vi "GenerateDGMLOwnerlessFilesFolderString.vi"(8 "Links in":T1, 9 "Nodes in":T1, 10 "ILabVIEWItem in":refnum<class "ILabVIEWItem.lvclass">, 11 "CGrapherDGML in":refnum<class "CGrapherDGML.lvclass">) -> (0 "Links":T1, 1 "Nodes":T1, 2 "Path":string="Z:\\OtherFiles", 3 "CGrapherDGML":refnum<class "CGrapherDGML.lvclass">)   [LabVIEW 2020, in "DefaultExtensions.lvlib" / "CGrapherDGML.lvclass"]
uses:
  CGrapherDGML.lvclass
  LabVIEWObjectInterfaces/ILabVIEWItem/ILabVIEWItem.lvclass
  LabVIEWItem/CLabVIEWItem/ConnectionSet.ctl
  CGrapherDGML.lvclass/CGrapherDGML.ctl
  ecf4d353-cf80-4459-a486-8bebc84a9ab0.vi
  LabVIEWItem/CLabVIEWItem/CLabVIEWItem.lvclass
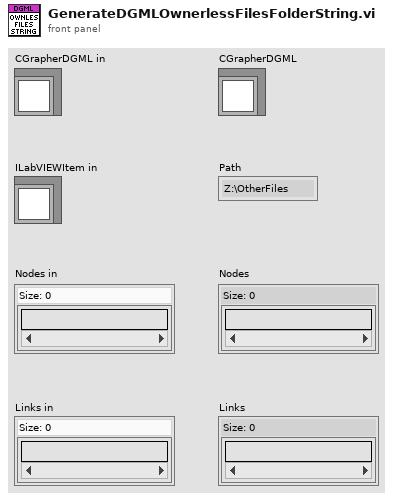
[diagram p1: front panel]
types:
  T1 = typedef "LabVIEWItem.lvlib/CLabVIEWItem.lvclass/ConnectionSet.ctl" = set{string}
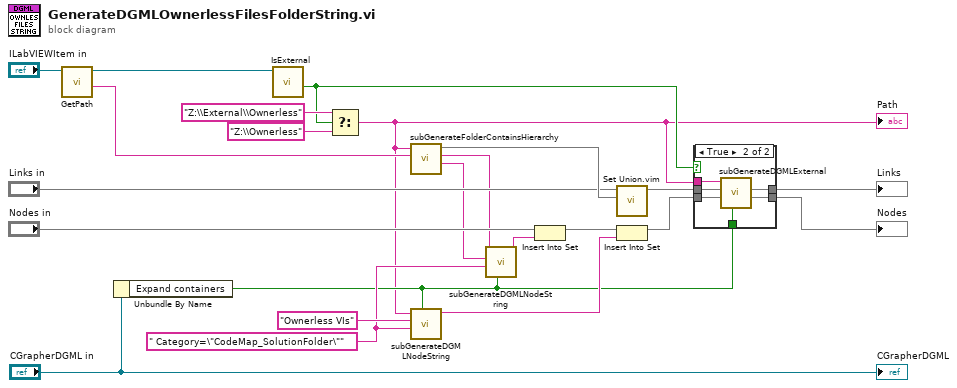
[diagram p0: block diagram]
diagram:
  w11 = " Category=\"CodeMap_SolutionFolder\"" ("format string")
  n1 = call-dynamic "GetPath.vi"("ILabVIEWItem in"="ILabVIEWItem in") -> ("Path"=w15:string, "ILabVIEWItem out"=w20:refnum<class "ILabVIEWItem.lvclass">)  [unwired: 8 in, 1 out]
  n2 = Unbundle By Name("CGrapherDGML in") -> ("Expand containers"=w3:bool)
  n3 = call-dynamic "IsExternal.vi"("ILabVIEWItem in"=w20) -> ("Is external?"=w2:bool)  [unwired: 8 in, 2 out]
  n4 = Select(t="Z:\\External\\Ownerless" ("format string"), s=w2, f="Z:\\Ownerless" ("format string")) -> (s? t:f=w1:string)
  "Path" <- w1
  n5 = call "subGenerateFolderContainsHierarchy.vi"("Path"=w15, "Source"=w1) -> ("Label"=w9:string, "New folder Id"=w10:string, "Links"=w23:T1)  [unwired: 7 in]
  n6 = call "subGenerateDGMLNodeString.vi"("Expand?"=w3, "Code schema"=w11, "Label"="Ownerless VIs" ("format string"), "Id"=w1) -> ("Node string"=w21:string)  [unwired: 7 in]
  n7 = call "subGenerateDGMLNodeString.vi"("Expand?"=w3, "Code schema"=w11, "Label"=w9, "Id"=w10) -> ("Node string"=w12:string)  [unwired: 7 in]
  n8 = Insert Into Set(10:w12, 11:"Nodes in") -> (3:w13:T1)  [unwired: 1 out]
  n9 = call "Set Union.vim"("set 2"=w23, "set 1"="Links in") -> ("union"=w7:T1)  [unwired: 9 in]
  n10 = Insert Into Set(10:w21, 11:w13) -> (3:w6:T1)  [unwired: 1 out]
  n11 = case shown="True" w2 {
    tunnel: w6 -> [w24 w31]
    tunnel: w7 -> [w25 w30]
    tunnel: w1 -> [_ w29]
    tunnel: w3 -> [_ w28]
    tunnel: [w25 w27] -> w5
    tunnel: [w24 w26] -> w4
    frame False {
    }
    frame True {
      n12 = call "subGenerateDGMLExternal.vi"("Expand?"=w28, "Nodes in in"=w31, "union in"=w30, "format string"=w29) -> ("Nodes out"=w26:T1, "union out"=w27:T1)  [unwired: 6 in]
    }
  }
  "Links" <- w5
  "Nodes" <- w4
  "CGrapherDGML" <- "CGrapherDGML in"
